vi "Get or Add SharedStringTablePart.vi"(8 "error in":errorcluster, 11 "SpreadsheetDoc in":refnum<k24>) -> (0 "error out":errorcluster, 2 "SharedStringTablePart":refnum<k24>, 3 "SpreadsheetDoc out":refnum<k24>)   [LabVIEW 2019, in "Open Xml.lvlib"]
uses:
  Open Xml.lvlib
  D:/git/Open-Xml-LabVIEW/Source/DocumentFormat.OpenXml.dll
  DocumentFormat.OpenXml.dll
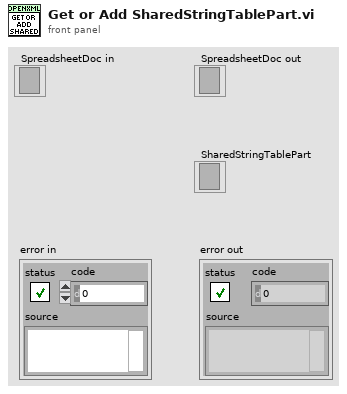
[diagram p1: front panel]
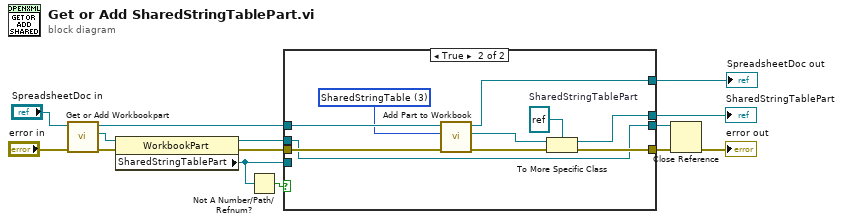
[diagram p0: block diagram]
diagram:
  n1 = call "Get or Add Workbookpart.vi"("error in"="error in", "SpreadsheetDoc in"="SpreadsheetDoc in") -> ("error out"=w8:errorcluster, "WorkbookPart"=w4:refnum<k24>, "SpreadsheetDoc out"=w2:refnum<k24>)  [unwired: 7 in]
  n2 = property class="WorkbookPart"(reference=w4, error in=w8) -> (reference out=w5:refnum<k24>, error out=w12:errorcluster, "SharedStringTablePart"=w11:refnum<k24>)
  n3 = Not A Number/Path/Refnum?(number/path/refnum=w11) -> (NaN/Path/Refnum?=w13:bool)
  n4 = case shown="True" w13 {
    tunnel: w5 -> [w16 w20]
    tunnel: w12 -> [w17 w23]
    tunnel: w11 -> [w18 _]
    tunnel: [w18 w27] -> w9
    tunnel: [w17 w26] -> w10
    tunnel: [w16 w20] -> w3
    tunnel: w2 -> [w15 w22]
    tunnel: [w15 w21] -> w1
    frame False {
    }
    frame True {
      w19 = 3 items=["Connections", "PivotTableCacheDefinition", "PivotTableCacheRecords", "SharedStringTable", "Worksheet", "WorkbookStyles"] ("PartType")
      w25 = refnum<k24> refnum  # SharedStringTablePart
      # "workbookPart.AddNewPart<SharedStringTablePart>();"
      n5 = call "Add Part to Workbook.vi"("error in"=w23, "PartType"=w19, "SpreadsheetDoc in"=w22) -> ("error out"=w24:errorcluster, "OpenXmlPart"=w28:refnum<k24>, "SpreadsheetDoc out"=w21:refnum<k24>)  [unwired: 6 in]
      n6 = To More Specific Class(target class=w25, reference=w28, error in=w24) -> (specific class reference=w27:refnum<k24>, error out=w26:errorcluster)
    }
  }
  "SharedStringTablePart" <- w9
  "SpreadsheetDoc out" <- w1
  n7 = Close Reference(reference=w3, error in (no error)=w10) -> (error out=→"error out":errorcluster)
